vi "ma_SML Power in Band.vi"(6 "impedance(ohm)":dbl=50.0 format="%.2f", 7 "units [rms]":T2(ring)=enum."V^2", 8 "error in (no error)":errorcluster, 9 "band":cluster{"center frequency":dbl, "bandwidth":dbl} {"bandwidth" format="%.2f"; "center frequency" format="%.2f"}, 10 "spectral info":T1 {"window" items=["Rectangle"=0, "Hanning"=1, "Hamming"=2, "Blackman-Harris"=3, "Exact Blackman"=4, "Blackman"=5, "Flat Top"=6, "4 Term B-Harris "=7, "7 Term B-Harris"=8, "Low Sidelobe"=9, "Blackman Nuttall"=11, "Triangle"=30, "Bartlett-Hanning"=31, "Bohman"=32, "Parzen"=33, "Welch"=34, "Kaiser"=60, "Dolph-Chebyshev"=61, "Gaussian"=62]}, 11 "power spectrum":T3 {"spectrum" format="%.2f"; "df" format="%.2f"; "f0" format="%.2f"}) -> (0 "error out":errorcluster, 2 "units string":string, 3 "power in band":dbl format="%.2f")   [LabVIEW 2020, in "NI_MAPro.lvlib"]
doc: "This VI calculates the power in band defined by <B>band</B> from the <B>Power Spectrum</B> input.\nThe input only takes unscaled <B>power spectrum</B>."
uses:
  NI_MAPro.lvlib
  ma_sml_Spectrum Cluster (real).ctl
  ma_sml_Spectral Info.ctl
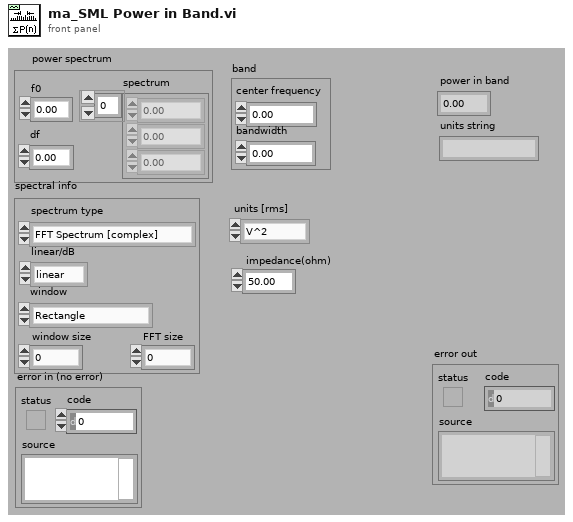
[diagram p1: front panel]
types:
  T1 = typedef "NI_MAPro.lvlib/ma_sml_Spectral Info.ctl" = cluster{"spectrum type":enum16{"FFT Spectrum [complex]", "Amplitude [Magnitude]", "Power [Magnitude^2]", "Cross Spectrum [complex]", "Frequency Response [Complex]"}, "linear/dB":enum16{"linear", "dB"}, "window":u16, "window size":i32, "FFT size":i32}
  T2 = enum16{"V", "V^2", "W", "dBm", "dBW", "dBV", "dBmV", "dBuV"}
  T3 = typedef "NI_MAPro.lvlib/ma_sml_Spectrum Cluster (real).ctl" = cluster{"f0":dbl, "df":dbl, "spectrum":dbl[]}
  T4 = enum16{"FFT Spectrum [complex]", "Amplitude [Magnitude]", "Power [Magnitude^2]", "Cross Spectrum [complex]", "Frequency Response [Complex]"}
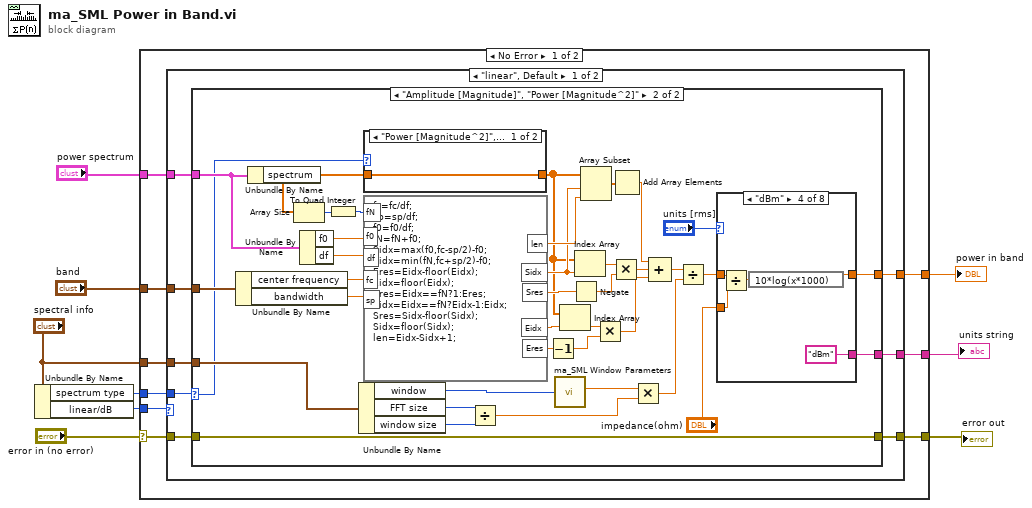
[diagram p0: block diagram]
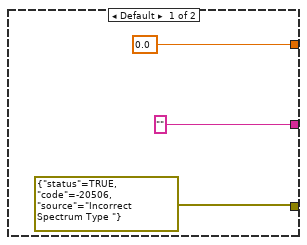
[diagram p2: hidden frame]
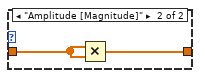
[diagram p3: hidden frame]
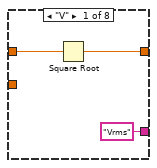
[diagram p4: hidden frame]
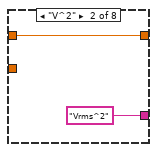
[diagram p5: hidden frame]
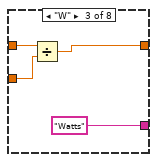
[diagram p6: hidden frame]
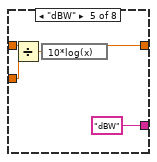
[diagram p7: hidden frame]
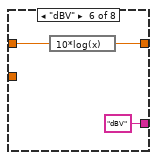
[diagram p8: hidden frame]
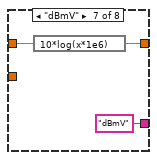
[diagram p9: hidden frame]
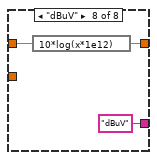
[diagram p10: hidden frame]
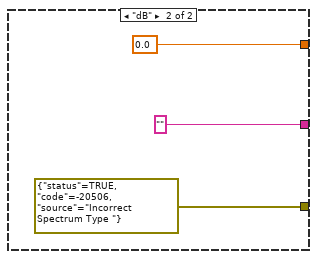
[diagram p11: hidden frame]
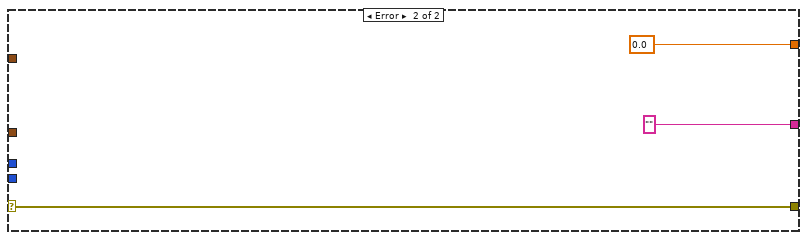
[diagram p12: hidden frame]
diagram:
  n1 = Unbundle By Name("spectral info") -> ("spectrum type"=w4:T4, "linear/dB"=w1:enum16{"linear", "dB"})
  n2 = case shown="No Error" "error in (no error)" {
    selector: "error in (no error)" -> [w10 w102]
    tunnel: "power spectrum" -> [w18 _]
    tunnel: "band" -> [w17 _]
    tunnel: [w16 "" ("Label")] -> w7
    tunnel: [w15 0.0] -> w6
    tunnel: [w14 w102] -> w5
    tunnel: w4 -> [w13 _]
    tunnel: "spectral info" -> [w12 _]
    tunnel: w1 -> [w11 _]
    frame No Error {
      n3 = case shown="\"linear\", Default" w11 {
        tunnel: w18 -> [w26 _]
        tunnel: w17 -> [w25 _]
        tunnel: [w24 "" ("Label")] -> w16
        tunnel: [w23 0.0] -> w15
        tunnel: w10 -> [w22 _]
        tunnel: [w21 errorcluster {"status"=TRUE, "code"=-20506, "source"="Incorrect Spectrum Type "} ("error in (no error)")] -> w14
        tunnel: w13 -> [w20 _]
        tunnel: w12 -> [w19 _]
        frame "linear", Default {
          n4 = case shown="\"Amplitude [Magnitude]\", \"Power [Magnitude^2]\"" w20 {
            selector: w20 -> [_ w31]
            tunnel: w26 -> [_ w45]
            tunnel: w25 -> [_ w44]
            tunnel: ["" ("Label") w43] -> w24
            tunnel: [0.0 w42] -> w23
            tunnel: w22 -> [_ w41]
            tunnel: [errorcluster {"status"=TRUE, "code"=-20506, "source"="Incorrect Spectrum Type "} ("error in (no error)") w41] -> w21
            tunnel: w19 -> [_ w40]
            frame Default {
            }
            frame "Amplitude [Magnitude]", "Power [Magnitude^2]" {
              n5 = Unbundle By Name(w44) -> ("center frequency"=w66:dbl, "bandwidth"=w65:dbl)
              n6 = Unbundle By Name(w45) -> ("spectrum"=w33:dbl[])
              n7 = Array Size(array=w33) -> (size(s)=w64:i32)
              n8 = Unbundle By Name(w45) -> ("f0"=w67:dbl, "df"=w63:dbl)
              n9 = To Quad Integer(1:w64) -> (0:w30:i64)
              n10 = Unbundle By Name(w40) -> ("window"=w37:u16, "FFT size"=w39:i32, "window size"=w38:i32)
              n11 = case shown="\"Power [Magnitude^2]\", Default" w31 {
                tunnel: [w68 w70] -> w32
                tunnel: w33 -> [w68 w69]
                frame "Power [Magnitude^2]", Default {
                }
                frame "Amplitude [Magnitude]" {
                  n12 = Multiply(x=w69, y=w69) -> (x*y=w70:dbl[])
                }
              }
              n13 = formula code="fc=fc/df;\nsp=sp/df;\nf0=f0/df;\nfN=fN+f0;\nSidx=max(f0,fc-sp/2)-f0;\nEidx=min(fN,fc+sp/2)-f0;\nEres=Eidx-floor(Eidx);\nEidx=floor(Eidx);\nEres=Eidx==fN?1:Eres;\nEidx=Eidx==fN?Eidx-1:Eidx;\nSres=Sidx-floor(Sidx);\nSidx=floor(Sidx);\nlen=Eidx-Sidx+1;"("f0"=w67, "df"=w63, "fc"=w66, "sp"=w65, "fN"=w30) -> ("Sidx"=w60:dbl, "Eidx"=w59:dbl, "len"=w62:dbl, "Eres"=w55:dbl, "Sres"=w57:dbl)
              n14 = Divide(x=w39, y=w38) -> (x/y=w35:dbl)
              n15 = Decrement(x=w55) -> (x-1=w46:dbl)
              n16 = call "ma_SML Window Parameters.vi"("window"=w37) -> ("ENBW"=w36:dbl)  [unwired: 3 out]
              n17 = Index Array(array=w32, index=w59) -> (element=w56:dbl)
              n18 = Negate(x=w57) -> (-x=w54:dbl)
              n19 = Index Array(array=w32, index=w60) -> (element=w58:dbl)
              n20 = Array Subset(array=w32, index=w60, length=w62) -> (w61:dbl[])
              n21 = Multiply(x=w56, y=w46) -> (x*y=w51:dbl)
              n22 = Multiply(x=w58, y=w54) -> (x*y=w52:dbl)
              n23 = Add Array Elements(numeric array=w61) -> (sum=w53:dbl)
              n24 = Multiply(x=w36, y=w35) -> (x*y=w34:dbl)
              n25 = Compound Arithmetic op=ADD(w53, w52, w51) -> (w50:dbl)
              n26 = Divide(x=w50, y=w34) -> (x/y=w48:dbl)
              n27 = case shown="\"dBm\"" "units [rms]" {
                tunnel: [w72 w75 w79 w80 w85 w91 w94 w97] -> w42
                tunnel: w48 -> [w73 w75 w78 w83 w89 w92 w95 w98]
                tunnel: "impedance(ohm)" -> [_ _ w77 w82 w88 _ _ _]
                tunnel: ["Vrms" ("Label") "Vrms^2" ("Label") "Watts" ("Label") "dBm" ("Label") "dBW" ("Label") "dBV" ("Label") "dBmV" ("Label") "dBuV" ("Label")] -> w43
                frame "V" {
                  n28 = Square Root(x=w73) -> (sqrt(x)=w72:dbl)
                }
                frame "V^2" {
                }
                frame "W" {
                  n29 = Divide(x=w78, y=w77) -> (x/y=w79:dbl)
                }
                frame "dBm" {
                  n30 = Divide(x=w83, y=w82) -> (x/y=w81:dbl)
                  n31 = expression code="10*log(x*1000)"(w81) -> (w80:dbl)
                }
                frame "dBW" {
                  n32 = Divide(x=w89, y=w88) -> (x/y=w86:dbl)
                  n33 = expression code="10*log(x)"(w86) -> (w85:dbl)
                }
                frame "dBV" {
                  n34 = expression code="10*log(x)"(w92) -> (w91:dbl)
                }
                frame "dBmV" {
                  n35 = expression code="10*log(x*1e6)"(w95) -> (w94:dbl)
                }
                frame "dBuV" {
                  n36 = expression code="10*log(x*1e12)"(w98) -> (w97:dbl)
                }
              }
            }
          }
        }
        frame "dB" {
        }
      }
    }
    frame Error {
    }
  }
  "error out" <- w5
  "power in band" <- w6
  "units string" <- w7
